vi "TestExec.Read Local Station Get SN From UUT Option.vi"(8 "error in":errorcluster, 11 "Config File Path":path) -> (0 "error out":errorcluster, 2 "Default Value":string, 3 "NotRequired":bool)   [LabVIEW 2018]
uses:
  <vilib>/Utility/config.llb/Read Key (String).vi
  <vilib>/Utility/config.llb/NI_LVConfig.lvlib
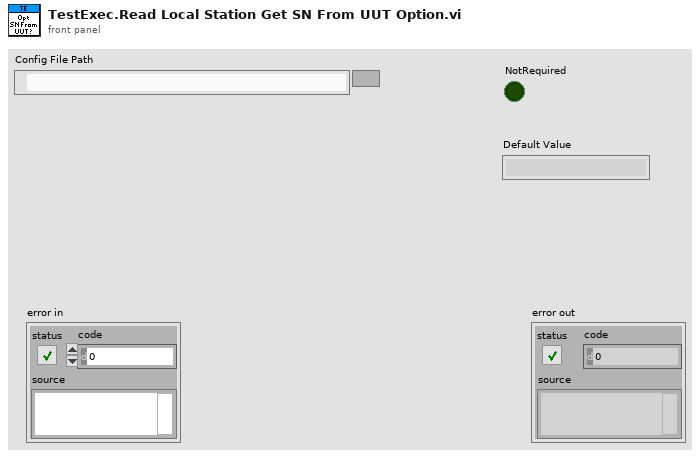
[diagram p1: front panel]
types:
  T1 = typedef "NI_LVConfig.lvlib/Config Data RefNum.ctl" = refnum<k1>
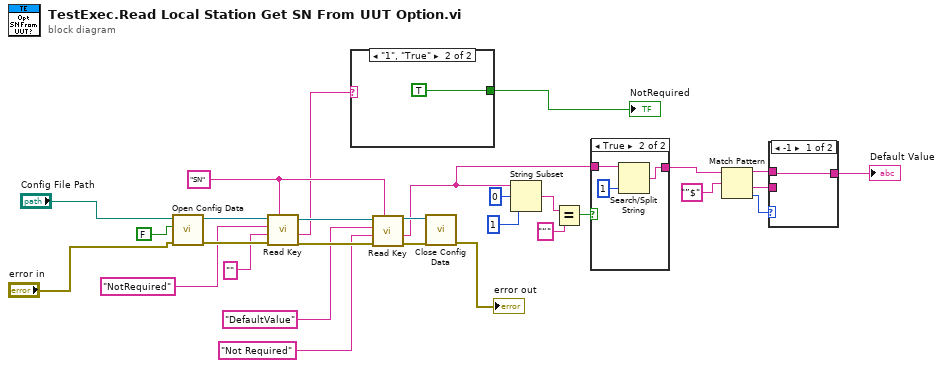
[diagram p0: block diagram]
diagram:
  w21 = "SN"
  n1 = call <vilib>:"Open Config Data.vi"("error in (no error)"="error in", "create file if necessary (T)"=FALSE, "configuration file path"="Config File Path") -> ("error out"=w27:errorcluster, "refnum"=w28:T1)  [unwired: 6 in, 1 out]
  n2 = call-poly <vilib>:"Read Key.vi"("section"=w21, "error in (no error)"=w27, "default value"="", "key"="NotRequired", "refnum"=w28) -> ("error out"=w20:errorcluster, "value"=w2:string, "refnum out"=w22:T1)  [unwired: 3 in, 1 out]
  n3 = case shown="\"1\", \"True\"" w2 {
    tunnel: [_ TRUE] -> w1
    frame "False", Default {
    }
    frame "1", "True" {
    }
  }
  "NotRequired" <- w1
  n4 = call-poly <vilib>:"Read Key.vi"("section"=w21, "error in (no error)"=w20, "default value"="Not Required", "key"="DefaultValue", "refnum"=w22) -> ("error out"=w19:errorcluster, "value"=w5:string, "refnum out"=w18:T1)  [unwired: 3 in, 1 out]
  n5 = call <vilib>:"Close Config Data.vi"("error in (no error)"=w19, "refnum"=w18) -> ("error out"=→"error out":errorcluster)  [unwired: 8 in, 1 out]
  n6 = String Subset(string=w5, offset (0)=0, length (rest)=1 ("length (rest)")) -> (substring=w8:string)
  n7 = Equal?(x=w8, y="“" ("regular expression (\"\")")) -> (x = y?=w6:bool)
  n8 = case shown="True" w6 {
    tunnel: w5 -> [w31 w34]
    tunnel: [w31 w32] -> w4
    frame False {
    }
    frame True {
      n9 = Search/Split String(string=w34, offset (0)=1) -> (match + rest of string=w32:string)  [unwired: 1 in, 2 out]
    }
  }
  n10 = Match Pattern(string=w4, regular expression="”$" ("regular expression (\"\")")) -> (before substring=w13:string, after substring=w12:string, offset past match=w14:i32)  [unwired: 1 in, 1 out]
  n11 = case shown="-1" w14 {
    tunnel: w13 -> [w35 w36]
    tunnel: w12 -> [_ _]
    tunnel: [w35 w36] -> w11
    frame -1 {
    }
    frame 0, Default {
    }
  }
  "Default Value" <- w11
